vi "GetRxData.vi"(6 "Tab data only(F)":bool=TRUE, 8 "error in (no error)":errorcluster, 11 "path":path) -> (0 "error out":errorcluster, 5 "dBFS/MHz":dbl[](array[numeric])=[-7.821, 19.941])   [LabVIEW 2018]
panel:
  out "standard output":string="2939 49c4\r\n403 6001\r\nFound COM4\r\nwr reg 0x02 0x0400\r\nwr reg 0x03 0x0000\r\nwr reg 0x04 1032\r\nwr reg 0x05 4\r\nwr reg 0x06 10\r\nwr reg 0x08 256\r\nwr reg 0x09 51\r\nwr reg 0x0A 4\r\nwr reg 0x0E 8000\r\nwr reg 0x0F 0x5555\r\nwr reg 0x10 0x0055\r\nwr reg 0x11 0xAAAA\r\nwr reg 0x12 0x00AA\r\nwr reg 0x1A 0x0000\r\nwr reg 0x1B 0x0000\r\nwr reg 0x17 0x0300\r\nwr reg 0x18 0x0000\r\nsos\r\nrd data\r\nMax Value: -7.821 dBFS at 19.941 MHz\r\n"
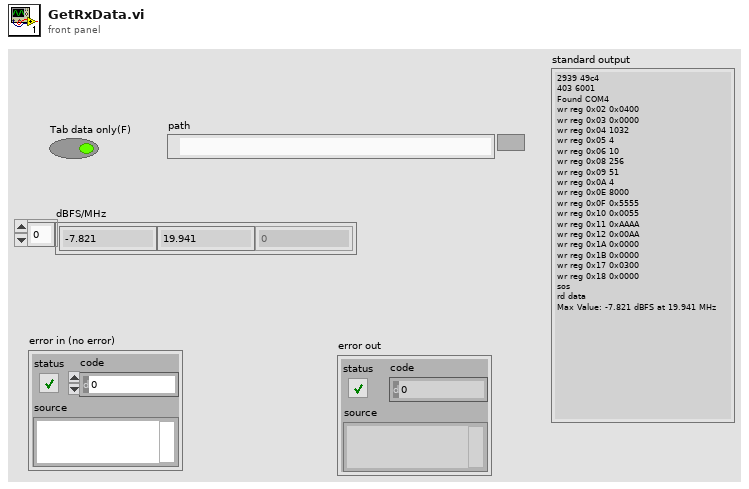
[diagram p1: front panel]
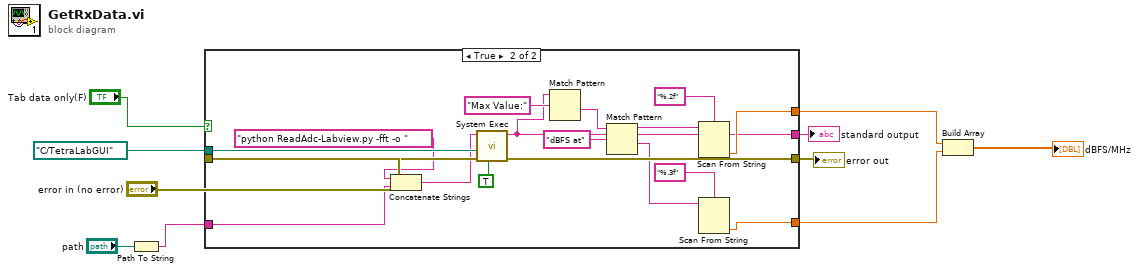
[diagram p0: block diagram]
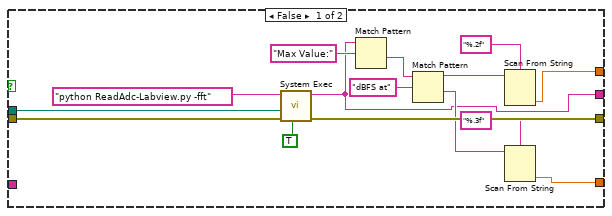
[diagram p2: hidden frame]
diagram:
  n1 = Path To String(path="path") -> (string=w2:string)
  n2 = case shown="True" "Tab data only(F)" {
    tunnel: path "C:/TetraLabGUI" ("working directory") -> [w25 w42]
    tunnel: [w11 w27] -> w3
    tunnel: "error in (no error)" -> [w23 w40]
    tunnel: [w22 w39] -> w7
    tunnel: [w13 w28] -> w5
    tunnel: [w12 w29] -> w4
    tunnel: w2 -> [_ w26]
    frame False {
      n3 = call <vilib>:"System Exec.vi"("run minimized? (F)"=TRUE, "error in (no error)"=w23, "working directory"=w25, "command line"="python ReadAdc-Labview.py -fft") -> ("error out"=w22:errorcluster, "standard output"=w11:string)  [unwired: 4 in, 2 out]
      n4 = Match Pattern(string=w11, regular expression="Max Value:") -> (after substring=w18:string)  [unwired: 1 in, 3 out]
      n5 = Match Pattern(string=w18, regular expression="dBFS at") -> (before substring=w19:string, after substring=w20:string)  [unwired: 1 in, 2 out]
      n6 = Scan From String(format string="%.2f", input string=w19) -> (output 1=w12:dbl)  [unwired: 3 in, 3 out]
      n7 = Scan From String(format string="%.3f", input string=w20) -> (output 1=w13:dbl)  [unwired: 3 in, 3 out]
    }
    frame True {
      n8 = Concatenate Strings("python ReadAdc-Labview.py -fft -o " ("command line"), w26) -> (w37:string)
      n9 = call <vilib>:"System Exec.vi"("run minimized? (F)"=TRUE, "error in (no error)"=w40, "working directory"=w42, "command line"=w37) -> ("error out"=w39:errorcluster, "standard output"=w27:string)  [unwired: 4 in, 2 out]
      n10 = Match Pattern(string=w27, regular expression="Max Value:") -> (after substring=w34:string)  [unwired: 1 in, 3 out]
      n11 = Match Pattern(string=w34, regular expression="dBFS at") -> (before substring=w35:string, after substring=w36:string)  [unwired: 1 in, 2 out]
      n12 = Scan From String(format string="%.2f", input string=w35) -> (output 1=w29:dbl)  [unwired: 3 in, 3 out]
      n13 = Scan From String(format string="%.3f", input string=w36) -> (output 1=w28:dbl)  [unwired: 3 in, 3 out]
    }
  }
  "error out" <- w7
  "standard output" <- w3
  n14 = Build Array(w4, w5) -> (→"dBFS/MHz":dbl[])
